vi "GetEnumStringValue.vi"(10 "Index":i32, 11 "Enum Variant":variant) -> (3 "string":string)   [LabVIEW 2013, in "JKI JSON Serialization.lvlib" / "JSON Serializer.lvclass"]
uses:
  JSON Serializer.lvclass
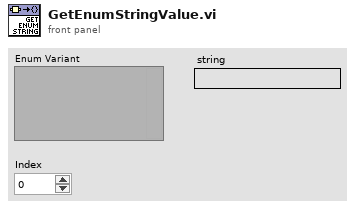
[diagram p1: front panel]
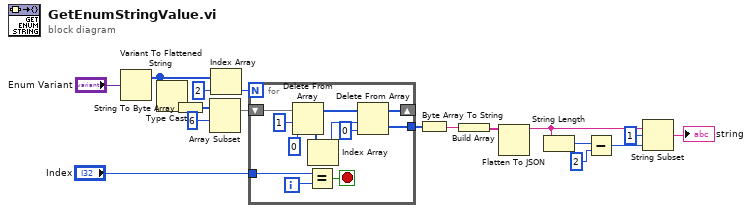
[diagram p0: block diagram]
diagram:
  n1 = Variant To Flattened String(Variant="Enum Variant") -> (1:w15:i16[])  [unwired: 1 out]
  n2 = Type Cast(x=w15) -> (*(type *) &x=w11:string)  [unwired: 1 in]
  n3 = String To Byte Array(string=w11) -> (unsigned byte array=w12:u8[])
  n4 = Array Subset(array=w12, index=6) -> (w13:u8[])  [unwired: 1 in]
  n5 = Index Array(array=w15, index=2) -> (element=w10:i16)
  n6 = for {
    N: w10 -> [_]
    shift-right: [w24] -> _
    shift-left: w13 -> [w30]
    tunnel: [w19] -> w9
    tunnel: "Index" -> [w21]
    i -> [w22]
    stop <- w20 stop-if-true
    n7 = Delete From Array(array=w30, length=1, index=0) -> (deleted portion=w27:u8[], array with subset deleted=w26:u8[])
    n8 = Equal?(x=w21, y=w22) -> (x = y?=w20:bool)
    n9 = Index Array(array=w27) -> (element=w25:u8)  [unwired: 1 in]
    n10 = Delete From Array(array=w26, length=w25, index=0) -> (deleted portion=w19:u8[], array with subset deleted=w24:u8[])
  }
  n11 = Byte Array To String(unsigned byte array=w9) -> (string=w3:string)
  n12 = Build Array(w3) -> (w8:string[])
  n13 = Flatten To JSON(anything=w8) -> (JSON string=w1:string)  [unwired: 2 in, 1 out]
  n14 = String Length(string=w1) -> (length=w6:i32)
  n15 = Subtract(x=w6, y=2) -> (x-y=w4:i32)
  n16 = String Subset(string=w1, offset (0)=1, length (rest)=w4) -> (substring=→"string":string)
